vi "FTW-Panel-DeferPanelUpdates.vi"(8 "error in":errorcluster, 10 "Defer?":bool=TRUE, 11 "VI Ref":refnum<vi>) -> (0 "error out":errorcluster, 3 "VI Ref out":refnum<vi>)   [LabVIEW 2015]
panel:
  # "Inputs"
  # "Outputs"
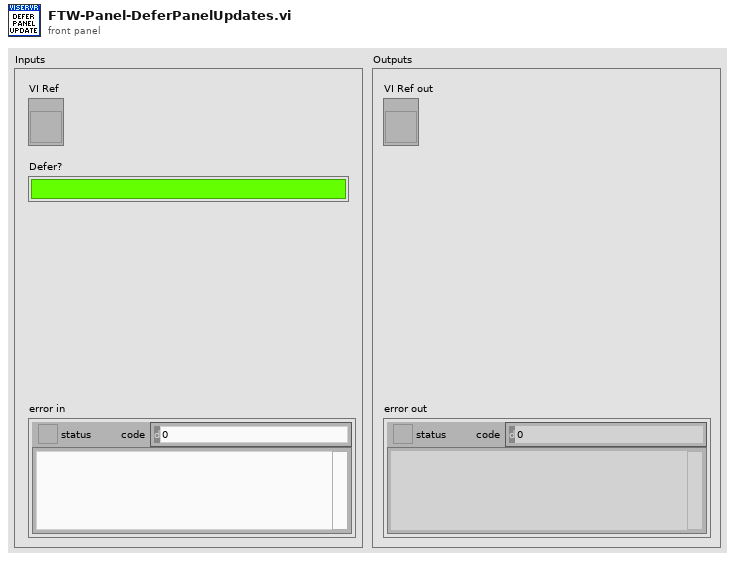
[diagram p1: front panel]
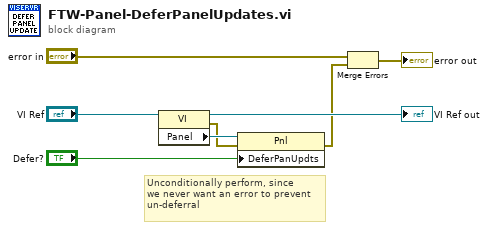
[diagram p0: block diagram]
diagram:
  # "Unconditionally perform, since\nwe never want an error to prevent\nun-deferral"
  n1 = property class="VI"(reference="VI Ref") -> (reference out=→"VI Ref out":refnum<vi>, error out=w5:errorcluster, "Panel"=w7:refnum<vi>)  [unwired: 1 in]
  n2 = property class="Pnl"(reference=w7, error in=w5, "DeferPanUpdts"="Defer?") -> (error out=w3:errorcluster)  [unwired: 1 out]
  n3 = Merge Errors("error in", w3) -> (→"error out":errorcluster)
